vi "TagArray to StarInputArray.vi"(7 "TagArray":refnum<class "Tag.lvclass">[](array[class]), 9 "error in (no error)":errorcluster) -> (8 "InputArray":T1(array[cluster]), 10 "error IO":errorcluster)   [LabVIEW 2014]
doc: "This VI converts an array of Tag objects to an array of Input clusters.\nInput is used for the input of Live Random Data to replace the current faulty working feedback node."
uses:
  Tag.lvclass
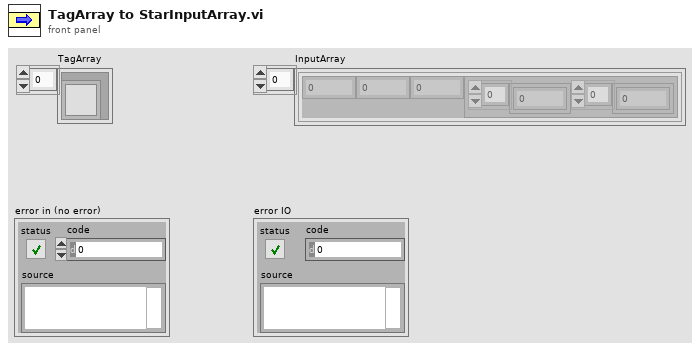
[diagram p1: front panel]
types:
  T1 = cluster{"TagID":dbl, "X":dbl, "Y":dbl, "AnchorIDDistanceCluster":cluster{"AnchorIDArray":dbl[], "AnchorDistanceArray":dbl[]}}[]
  T2 = cluster{"AnchorIDArray":dbl[], "AnchorDistanceArray":dbl[]}
  T3 = cluster{"Tag ID":dbl, "TagX":dbl, "TagY":dbl, "AnchorIDDistanceCluster":cluster{"AnchorIDArray":dbl[], "AnchorDistanceArray":dbl[]}}
  T4 = cluster{"Tag ID":dbl, "TagX":dbl, "TagY":dbl, "AnchorIDDistanceCluster":cluster{"AnchorIDArray":dbl[], "AnchorDistanceArray":dbl[]}}[]
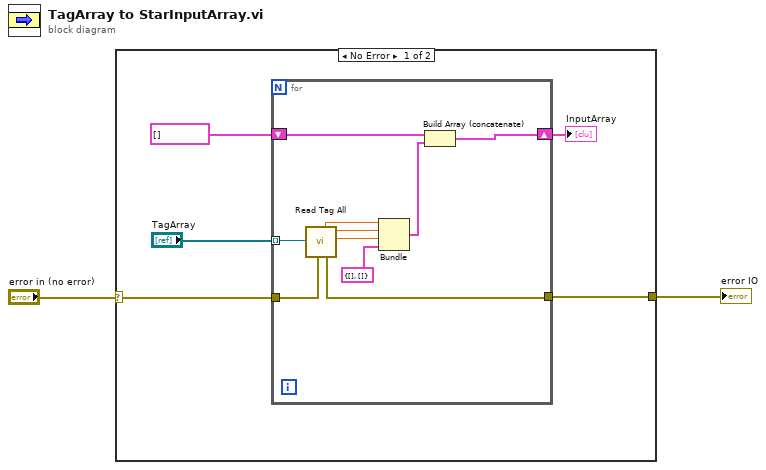
[diagram p0: block diagram]
diagram:
  n1 = case shown="No Error" "error in (no error)" {
    selector: "error in (no error)" -> [w4 w18]
    tunnel: [w3 w18] -> w1
    frame No Error {
      n2 = for {
        tunnel: "TagArray" -> [w17] mode=indexing
        shift-right: [w10] -> w5
        shift-left: T1 [] ("InputArrayConstant") -> [w12]
        tunnel: w4 -> [w9]
        tunnel: [w8] -> w3
        n3 = call "Read Tag All.vi"("error in (no error)"=w9, "Tag.lvclass"=w17) -> ("TagY"=w14:dbl, "TagX"=w15:dbl, "error out"=w8:errorcluster, "Tag ID"=w16:dbl)  [unwired: 4 in, 2 out]
        n4 = Bundle("Tag ID"=w16, "TagX"=w15, "TagY"=w14, "AnchorIDDistanceCluster"=T2 {"AnchorIDArray"=[], "AnchorDistanceArray"=[]}) -> (w11:T3)  [unwired: 1 in]
        n5 = Build Array (concatenate)(w12, w11) -> (w10:T4)
      }
      "InputArray" <- w5
    }
    frame Error {
    }
  }
  "error IO" <- w1
